vi "DHE_LoadIIDs.vi"(8 "error in (no error)":errorcluster) -> (0 "error out":errorcluster, 1 "autoid":string="LASTIMG", 2 "expidbase":string="LASTIMG", 4 "expidcounter":i32)   [LabVIEW 2016]
uses:
  <vilib>/Utility/config.llb/Read Key (String).vi
  <vilib>/Utility/config.llb/Read Key (I32).vi
  <vilib>/Utility/config.llb/NI_LVConfig.lvlib
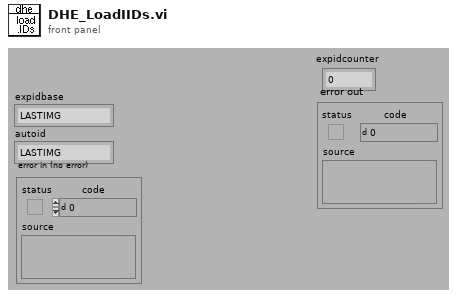
[diagram p1: front panel]
types:
  T1 = typedef "NI_LVConfig.lvlib/Config Data RefNum.ctl" = refnum<k1>
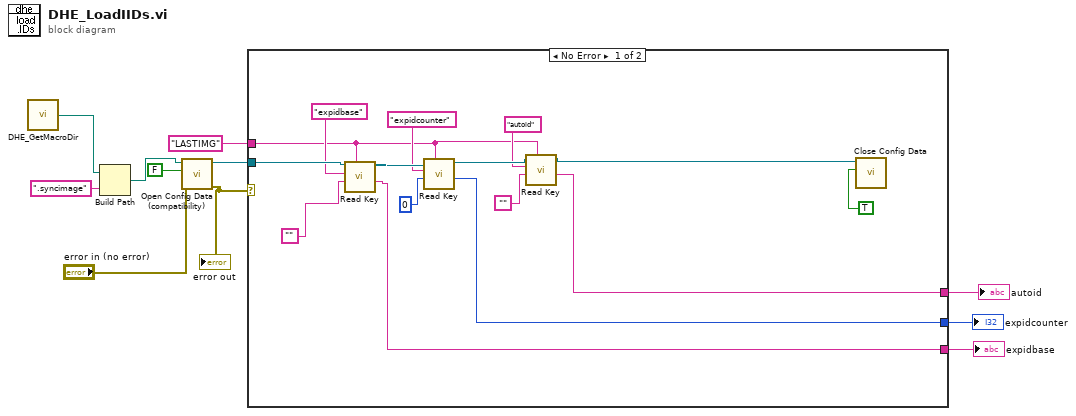
[diagram p0: block diagram]
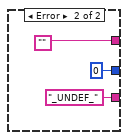
[diagram p2: hidden frame]
diagram:
  n1 = call "DHE_GetMacroDir.vi"() -> ("DHE_MacroDir"=w6:path)  [unwired: 9 out]
  n2 = Build Path(base path=w6, name or relative path=".syncimage") -> (appended path=w7:path)
  n3 = call <vilib>:"Open Config Data (compatibility).vi"("error in (no error)"="error in (no error)", "create file if necessary (T)"=FALSE ("create file if necessary? (T)"), "configuration file path"=w7) -> ("error out"=w5:errorcluster, "refnum"=w11:T1)  [unwired: 6 in, 1 out]
  "error out" <- w5
  n4 = case shown="No Error" w5 {
    tunnel: w11 -> [w26 _]
    tunnel: "LASTIMG" ("section") -> [w13 _]
    tunnel: [w21 "_UNDEF_" ("value")] -> w4
    tunnel: [w18 0 ("value")] -> w3
    tunnel: [w15 ""] -> w2
    frame No Error {
      n5 = call-poly <vilib>:"Read Key.vi"("section"=w13, "default value"="", "key"="expidbase", "refnum"=w26) -> ("value"=w21:string, "refnum out"=w25:T1)  [unwired: 2 in, 4 out]
      n6 = call-poly <vilib>:"Read Key.vi"("section"=w13, "default value"=0 ("number"), "key"="expidcounter", "refnum"=w25) -> ("value"=w18:i32, "refnum out"=w23:T1)  [unwired: 1 in, 5 out]
      n7 = call-poly <vilib>:"Read Key.vi"("section"=w13, "default value"="", "key"="autoid", "refnum"=w23) -> ("value"=w15:string, "refnum out"=w12:T1)  [unwired: 2 in, 4 out]
      n8 = call <vilib>:"Close Config Data.vi"("write file if changed (T)"=TRUE ("write configuration file? (F)"), "refnum"=w12) -> ()  [unwired: 1 in, 9 out]
    }
    frame Error {
    }
  }
  "expidbase" <- w4
  "expidcounter" <- w3
  "autoid" <- w2
